vi "题目二.vi"() -> ()   [LabVIEW 2017]
uses:
  <vilib>/Waveform/WDTFileIO.llb/ Write Waveform to File.vi
  <vilib>/Waveform/WDTFileIO.llb/Read Waveform from File.vi
  <vilib>/measure/NI_MABase.lvlib
panel:
  out "all waveforms in record":waveform(dbl)[](array[waveform]) caption="记录中所有波形"
  out "波形图表":waveform(dbl)[](graph)
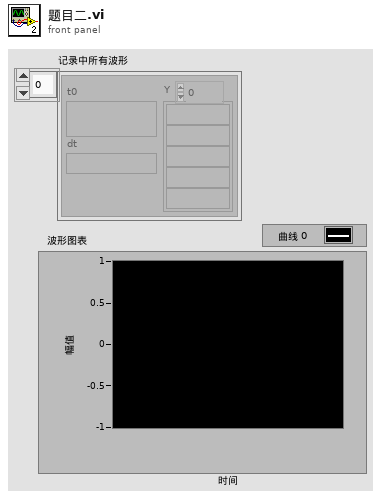
[diagram p1: front panel]
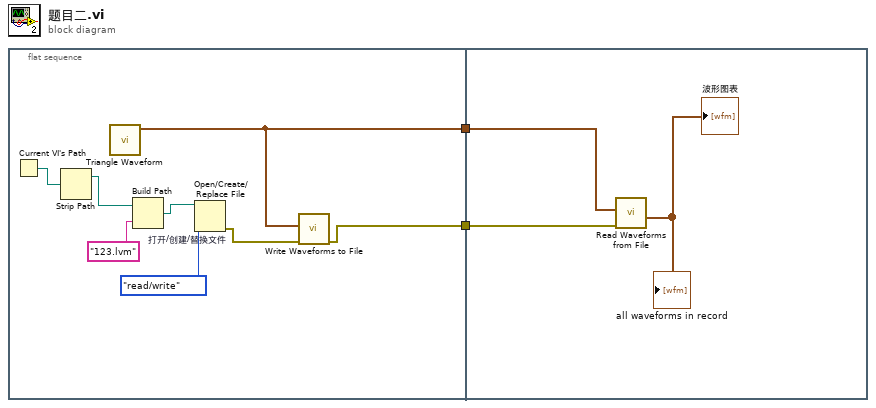
[diagram p0: block diagram]
diagram:
  n1 = flat-sequence {
    tunnel: [w4] -> w2
    tunnel: [w3] -> w1
    tunnel: w2 -> [w13]
    tunnel: w1 -> [w12]
    frame #0 {
      n2 = Current VI's Path() -> (path=w10:path)
      n3 = Strip Path(path=w10) -> (stripped path=w9:path)  [unwired: 1 out]
      n4 = call <vilib>:"Triangle Waveform.vi"() -> ("signal out"=w4:waveform(dbl))  [unwired: 10 in, 1 out]
      n5 = Build Path(base path=w9, name or relative path="123.lvm") -> (appended path=w5:path)
      n6 = Open/Create/Replace File "打开/创建/替换文件"(file path (use dialog)=w5, access (0:read/write)=enum16{"read/write", "read-only", "write-only"}."read/write" ("权限(0:read/write)")) -> (error out=w6:errorcluster)  [unwired: 4 in, 2 out]
      n7 = call-poly <vilib>:"Write Waveforms to File.vi"("error in (no error)"=w6, "waveform"=w4) -> ("error out"=w3:errorcluster)  [unwired: 8 in, 1 out]
    }
    frame #1 {
      n8 = call-poly <vilib>:"Read Waveforms from File.vi"("error in (no error)"=w12, "offset (records:0)"=w13) -> ("all waveforms in record"=→"波形图表" →"all waveforms in record":waveform(dbl)[])  [unwired: 4 in, 3 out]
    }
  }
